vi "Beam Break Control.vi"(2 "Variables":string[](array[string]), 3 "SRE":T1) -> (0 "Value":bool)   [LabVIEW 2014]
uses:
  TypeDefs/SRE Enum.ctl
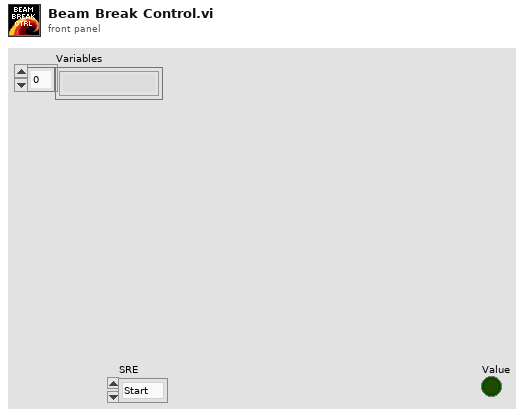
[diagram p1: front panel]
types:
  T1 = typedef "SRE Enum.ctl" = enum16{"Start", "Run", "End"}
  T2 = typedef "WPI_DigitalInputDevRef.ctl" = cluster{"DevStatus":errorcluster, "DIO Channel":T3, "Controller":T4}
  T3 = typedef "FPGA_DIOChannel.ctl" = enum8{"DIO 0", "DIO 1", "DIO 2", "DIO 3", "DIO 4", "DIO 5", "DIO 6", "DIO 7", "DIO 8", "DIO 9", "DIO MXP 0", "DIO MXP 1", "DIO MXP 2", "DIO MXP 3", "DIO MXP 4", "DIO MXP 5", "DIO MXP 6", "DIO MXP 7", "DIO MXP 8", "DIO MXP 9", "DIO MXP 10", "DIO MXP 11", "DIO MXP 12", "DIO MXP 13", "DIO MXP 14", "DIO MXP 15", "Invalid"}
  T4 = typedef "FPGA_TypedefDigitalModule.ctl" = enum16{"Controller 1"}
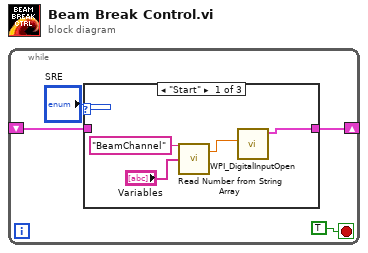
[diagram p0: block diagram]
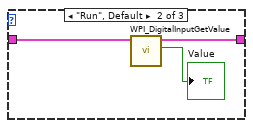
[diagram p2: hidden frame]
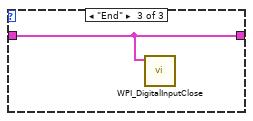
[diagram p3: hidden frame]
diagram:
  n1 = while {
    shift-right: [w3] -> _
    shift-left: _ -> [w2]
    stop <- TRUE stop-if-true
    n2 = case shown="\"Start\"" "SRE" {
      tunnel: [w8 w10 w12] -> w3
      tunnel: w2 -> [_ w11 w12]
      frame "Start" {
        n3 = call "Read Number from String Array.vi"("Variables"="Variables", "Name"="BeamChannel") -> ("number"=w6:dbl)  [unwired: 1 in, 1 out]
        n4 = call <vilib>:"WPI_DigitalInputOpen.vi"("DIO Channel"=w6) -> ("DigitalInputDevRef"=w8:T2)  [unwired: 9 in, 1 out]
      }
      frame "Run", Default {
        n5 = call <vilib>:"WPI_DigitalInputGetValue.vi"("DigitalInputDevRef"=w11) -> ("Value"=→"Value":bool, "DigitalInputDevRef"=w10:T2)  [unwired: 8 in, 1 out]
      }
      frame "End" {
        n6 = call <vilib>:"WPI_DigitalInputClose.vi"("DigitalInputDevRef"=w12) -> ()  [unwired: 10 in, 1 out]
      }
    }
  }
